vi "set_settings_cluster.vi"(8 "error in (no error)":errorcluster, 10 "settings cluster variant":variant, 11 "DataCollectionDL090215 in":refnum<class "DataCollectionDL090215.lvclass">) -> (0 "error out":errorcluster, 3 "DataCollectionDL090215 out":refnum<class "DataCollectionDL090215.lvclass">)   [LabVIEW 2010, in "DataCollectionDL090215.lvclass"]
uses:
  DataCollectionDL090215.lvclass
  DataCollectionDL090215.lvclass/DataCollectionDL090215.ctl
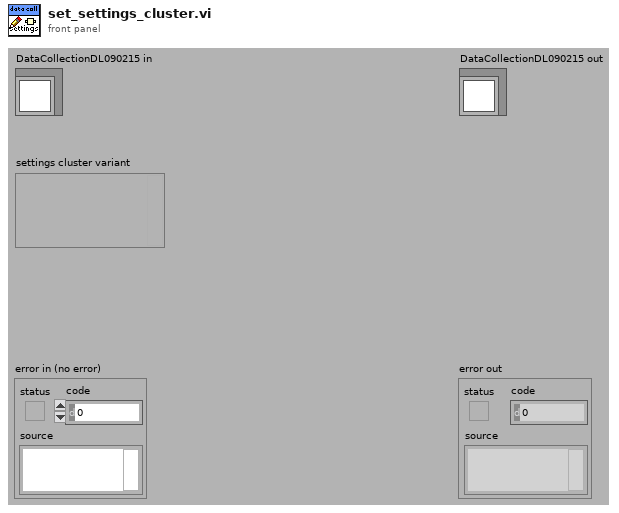
[diagram p1: front panel]
types:
  T1 = typedef "DataCollectionDL090215.lvclass/settings_cluster.ctl" = cluster{"saving":cluster{"autosave?":bool, "write header?":bool, "channels to save":bool[]}, "shared variables":cluster{"notebook import string ref":refnum<k21>, "OME header import string ref":refnum<k21>}}
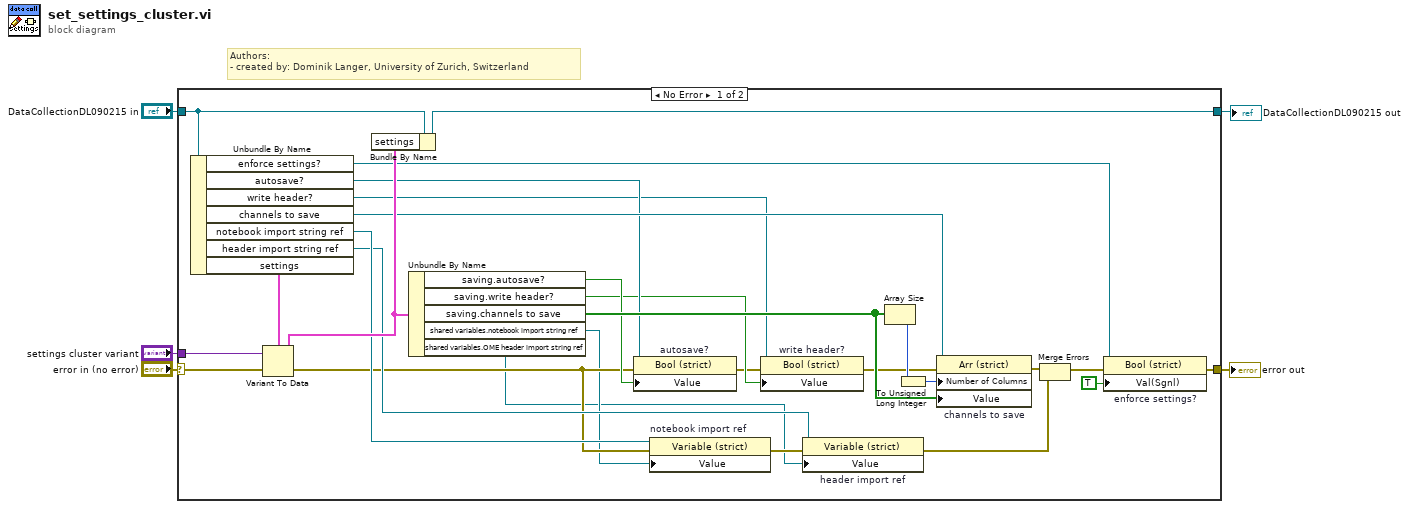
[diagram p0: block diagram]
diagram:
  # "Authors: \n- created by: Dominik Langer, University of Zurich, Switzerland"
  n1 = case shown="No Error" "error in (no error)" {
    selector: "error in (no error)" -> [w33 w35]
    tunnel: "settings cluster variant" -> [w31 _]
    tunnel: "DataCollectionDL090215 in" -> [w30 w34]
    tunnel: [w7 w35] -> w2
    tunnel: [w29 w34] -> w1
    frame No Error {
      n2 = Unbundle By Name(w30) -> ("enforce settings?"=w9:refnum<vi>, "autosave?"=w23:refnum<vi>, "write header?"=w22:refnum<vi>, "channels to save"=w27:refnum<vi>, "notebook import string ref"=w16:refnum<vi>, "header import string ref"=w15:refnum<vi>, "settings"=w32:T1)
      n3 = Variant To Data(error in=w33, Variant=w31, type=w32) -> (error out=w12:errorcluster, data=w28:T1)
      n4 = Bundle By Name(cluster=w30, "settings"=w28) -> (w29:refnum<class "DataCollectionDL090215.lvclass">)
      n5 = Unbundle By Name(w28) -> ("saving.autosave?"=w21:bool, "saving.write header?"=w20:bool, "saving.channels to save"=w24:bool[], "shared variables.notebook import string ref"=w11:refnum<k21>, "shared variables.OME header import string ref"=w10:refnum<k21>)
      n6 = property on="autosave?" class="Bool (strict)"(reference=w23, error in=w12, "Value"=w21) -> (error out=w19:errorcluster)  [unwired: 1 out]
      n7 = property on="notebook import ref" class="Variable (strict)"(reference=w16, error in=w12, "Value"=w11) -> (error out=w17:errorcluster)  [unwired: 1 out]
      n8 = property on="write header?" class="Bool (strict)"(reference=w22, error in=w19, "Value"=w20) -> (error out=w18:errorcluster)  [unwired: 1 out]
      n9 = property on="header import ref" class="Variable (strict)"(reference=w15, error in=w17, "Value"=w10) -> (error out=w14:errorcluster)  [unwired: 1 out]
      n10 = Array Size(array=w24) -> (size(s)=w26:i32)
      n11 = To Unsigned Long Integer(number=w26) -> (unsigned 32bit integer=w25:u32)
      n12 = property on="channels to save" class="Arr (strict)"(reference=w27, error in=w18, "Number of Columns"=w25, "Value"=w24) -> (error out=w13:errorcluster)  [unwired: 1 out]
      n13 = Merge Errors(w13, w14) -> (w8:errorcluster)
      n14 = property on="enforce settings?" class="Bool (strict)"(reference=w9, error in=w8, "Val(Sgnl)"=TRUE ("Value (Signaling)")) -> (error out=w7:errorcluster)  [unwired: 1 out]
    }
    frame Error {
    }
  }
  "error out" <- w2
  "DataCollectionDL090215 out" <- w1
